vi "Configure AC Volts.vi"(0 "VISA resource name":refnum<visa-resource-name>, 5 "error in (no error)":errorcluster, 6 "Auto Range? (T: Auto)":bool=TRUE, 7 "Digital Filter (0: Off)":u16(ring) items=["Off", "Moving Filter", "Repeating Filter"], 8 "Custom Range (100mV)":dbl=0.1 min=0.1 max=750.0 format="%#.6e", 9 "Digital Filter Readings (10)":i32=10, 10 "Function":i32(ring) items=["Primary", "Secondary"], 11 "Bandwidth (20 Hz)":i32(ring)=1 items=["3 Hz ~ 300 KHz", "20 Hz ~ 300 KHz", "200 Hz ~ 300 KHz"]) -> (14 "VISA resource name out":refnum<visa-resource-name>, 19 "error out":errorcluster)   [LabVIEW 2024, in "Keithley 2100 Series.lvlib"]
doc: "This VI configures the instrument to measure AC Volts."
uses:
  Keithley 2100 Series.lvlib
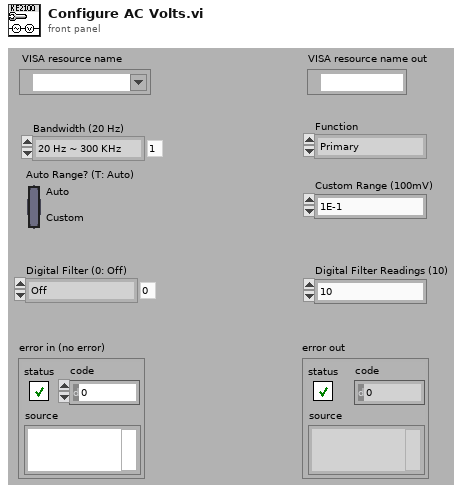
[diagram p1: front panel]
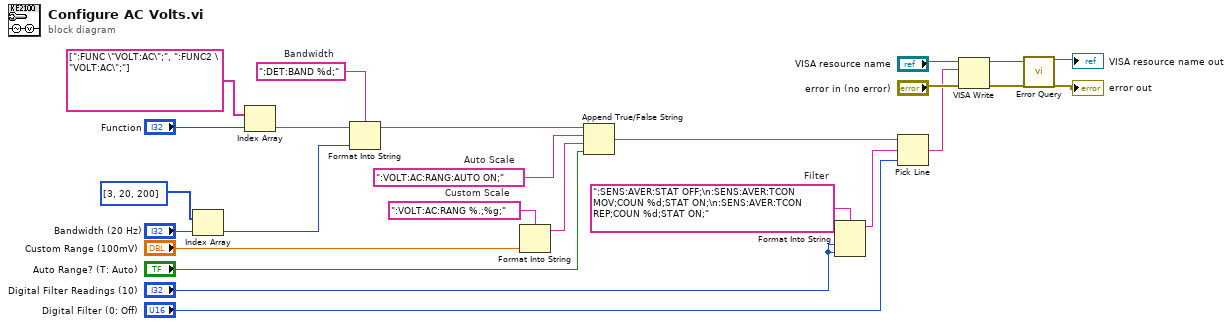
[diagram p0: block diagram]
diagram:
  w17 = ":SENS:AVER:STAT OFF;\n:SENS:AVER:TCON MOV;COUN %d;STAT ON;\n:SENS:AVER:TCON REP;COUN %d;STAT ON;"  # Filter
  w20 = ":VOLT:AC:RANG:AUTO ON;"  # Auto Scale
  w22 = ":VOLT:AC:RANG %.;%g;"  # Custom Scale
  w23 = ":DET:BAND %d;"  # Bandwidth
  n1 = Index Array(array=i32[] [3, 20, 200], index="Bandwidth (20 Hz)") -> (element=w4:i32)
  n2 = Index Array(array=string[] [":FUNC \"VOLT:AC\";", ":FUNC2 \"VOLT:AC\";"], index="Function") -> (element=w1:string)
  n3 = Format Into String(format string=w23, initial string=w1, w4) -> (resulting string=w10:string)  [unwired: 1 in, 1 out]
  n4 = Format Into String(format string=w22, "Custom Range (100mV)") -> (resulting string=w21:string)  [unwired: 2 in, 1 out]
  n5 = Append True/False String(1:"Auto Range? (T: Auto)", 2:w21, 3:w20, 4:w10) -> (0:w13:string)
  n6 = Format Into String(format string=w17, "Digital Filter Readings (10)", "Digital Filter Readings (10)") -> (resulting string=w18:string)  [unwired: 2 in, 1 out]
  n7 = Pick Line(string ("")=w13, multi-line string=w18, line index="Digital Filter (0: Off)") -> (output string=w7:string)
  n8 = VISA Write(VISA resource name="VISA resource name", write buffer=w7, error in (no error)="error in (no error)") -> (VISA resource name out=w12:refnum<visa-resource-name>, error out=w11:errorcluster)  [unwired: 1 out]
  n9 = call "Error Query.vi"("VISA resource name"=w12, "error in (no error)"=w11) -> ("VISA resource name out"=→"VISA resource name out":refnum<visa-resource-name>, "error out"=→"error out":errorcluster)  [unwired: 14 in, 2 out]
